vi "Humidity.vi"(1 "Variable name":string, 2 "Chaîne":string) -> (0 "Numeric":dbl)   [LabVIEW 2018]
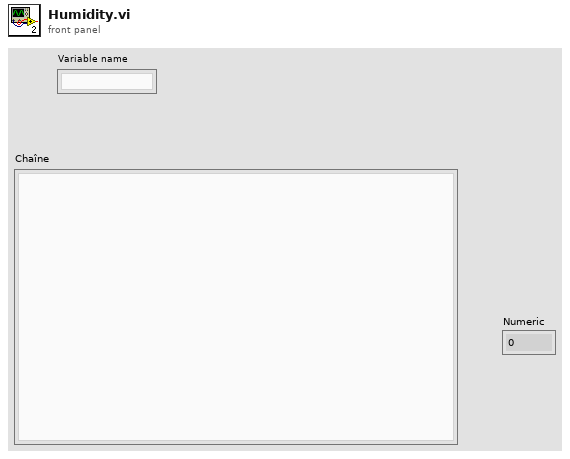
[diagram p1: front panel]
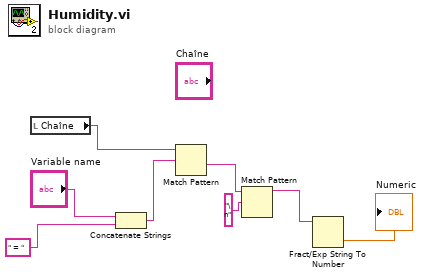
[diagram p0: block diagram]
diagram:
  n1 = local read "Chaîne"() -> (w1:string)
  n2 = Concatenate Strings("Variable name", " = " ("regular expression")) -> (w5:string)
  n3 = Match Pattern(string=w1, regular expression=w5) -> (after substring=w4:string)  [unwired: 1 in, 3 out]
  n4 = Match Pattern(string=w4, regular expression="\n") -> (before substring=w3:string)  [unwired: 1 in, 3 out]
  n5 = Fract/Exp String To Number(string=w3) -> (number=→"Numeric":dbl)  [unwired: 3 in, 1 out]
